vi "ODrive State and Info.vi"() -> ()   [LabVIEW 2016, in "Shared resources RT.lvlib"]
uses:
  Shared resources RT.lvlib
panel:
  out "ODrive State":u8
  out "ODrive Errors":u32
  out "ODrive Error Flags":bool[](array[boolean])
  out "Position Axis1":i16
  out "Velocity Axis0":i16
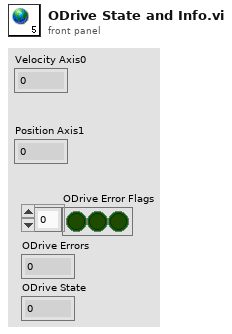
[diagram p1: front panel]
diagram:
